vi "Populate Tree.vi"(0 "TreeControl in":refnum<vi>, 5 "VI list":T1[](array[typedef]), 7 "Folder list":T1[](array[typedef]), 11 "error in (no error)":errorcluster) -> (4 "TreeControl out":refnum<vi>, 15 "error out":errorcluster)   [LabVIEW 2021, in "Migrator.lvlib"]
uses:
  Migrator.lvlib
  controls/Multiple Migration/Tree Items.ctl
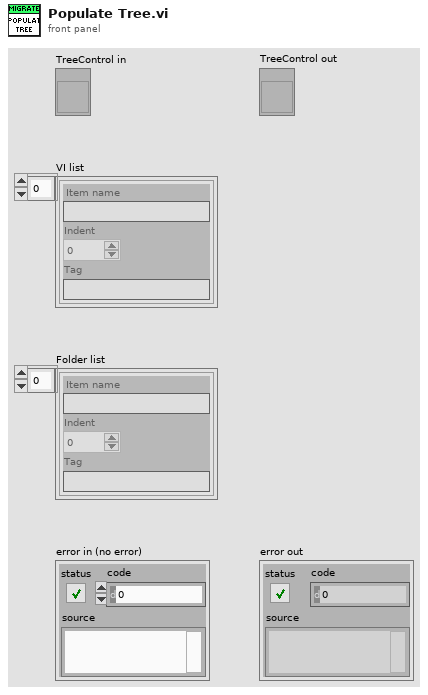
[diagram p1: front panel]
types:
  T1 = typedef "Migrator.lvlib/Tree Items.ctl" = cluster{"Item name":string, "Indent":i32, "Tag":string}
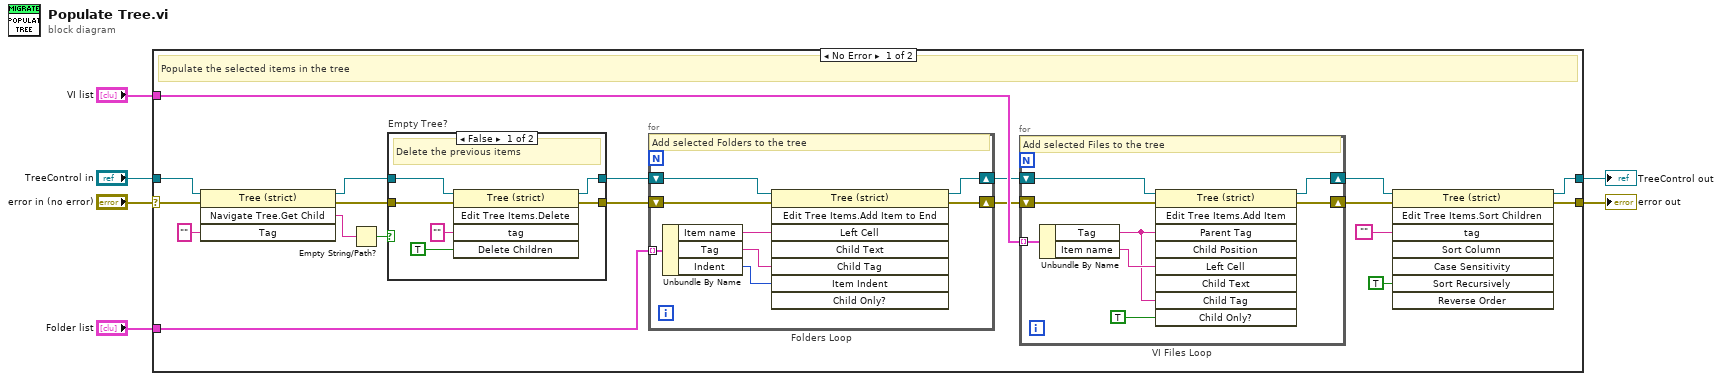
[diagram p0: block diagram]
diagram:
  n1 = case shown="No Error" "error in (no error)" {
    selector: "error in (no error)" -> [w13 w51]
    tunnel: [w22 w51] -> w6
    tunnel: "TreeControl in" -> [w11 w50]
    tunnel: "VI list" -> [w24 _]
    tunnel: "Folder list" -> [w16 _]
    tunnel: [w21 w50] -> w1
    frame No Error {
      # "Populate the selected items in the tree"
      n2 = invoke class="Tree (strict)" method="Navigate Tree.Get Child"(reference=w11, error in=w13, "Tag"="") -> (reference out=w7:refnum<vi>, error out=w12:errorcluster, "Navigate Tree:Get Child"=w9:string)  [unwired: 1 in, 1 out]
      n3 = Empty String/Path?(string/path=w9) -> (empty?=w8:bool)
      n4 = case "Empty Tree?" shown="False" w8 {
        tunnel: [w31 w32] -> w18
        tunnel: [w30 w33] -> w17
        tunnel: w12 -> [w27 w32]
        tunnel: w7 -> [w26 w33]
        frame False {
          # "Delete the previous items"
          n5 = invoke class="Tree (strict)" method="Edit Tree Items.Delete"(reference=w26, error in=w27, "tag"="" ("Tag"), "Delete Children"=TRUE ("Delete Children?")) -> (reference out=w30:refnum<vi>, error out=w31:errorcluster)  [unwired: 1 in, 3 out]
        }
        frame True {
          # "Pass"
        }
      }
      n6 = for "Folders Loop" {
        shift-right: [w48] -> w23
        shift-left: w18 -> [w49]
        shift-right: [w46] -> w15
        shift-left: w17 -> [w47]
        tunnel: w16 -> [w45] mode=indexing
        # "Add selected Folders to the tree"
        n7 = Unbundle By Name(w45) -> ("Item name"=w44:string, "Tag"=w43:string, "Indent"=w42:i32)
        n8 = invoke class="Tree (strict)" method="Edit Tree Items.Add Item to End"(reference=w47, error in=w49, "Left Cell"=w44, "Child Tag"=w43, "Item Indent"=w42) -> (reference out=w46:refnum<vi>, error out=w48:errorcluster)  [unwired: 3 in, 6 out]
      }
      n9 = for "VI Files Loop" {
        shift-right: [w39] -> w25
        shift-left: w23 -> [w38]
        tunnel: w24 -> [w41] mode=indexing
        shift-right: [w34] -> w14
        shift-left: w15 -> [w35]
        # "Add selected Files to the tree"
        n10 = Unbundle By Name(w41) -> ("Tag"=w36:string, "Item name"=w40:string)
        n11 = invoke class="Tree (strict)" method="Edit Tree Items.Add Item"(reference=w35, error in=w38, "Parent Tag"=w36, "Left Cell"=w40, "Child Tag"=w36, "Child Only?"=TRUE) -> (reference out=w34:refnum<vi>, error out=w39:errorcluster)  [unwired: 3 in, 7 out]
      }
      n12 = invoke class="Tree (strict)" method="Edit Tree Items.Sort Children"(reference=w14, error in=w25, "tag"="", "Sort Recursively"=TRUE ("Sort Recursively?")) -> (reference out=w21:refnum<vi>, error out=w22:errorcluster)  [unwired: 4 in, 6 out]
    }
    frame Error {
      # "Pass"
    }
  }
  "error out" <- w6
  "TreeControl out" <- w1
